vi "GetPanes.vi"(6 "error in":errorcluster, 9 "VI Interpreter in":refnum<class "VI Interpreter.lvclass">) -> (0 "error out":errorcluster, 3 "VI Interpreter out":refnum<class "VI Interpreter.lvclass">, 4 "Panes":refnum<class "Pane.lvclass">[](array[class]))   [LabVIEW 2014, in "VI Interpreter.lvclass"]
uses:
  VI Interpreter.lvclass
  Pane/Pane.lvclass
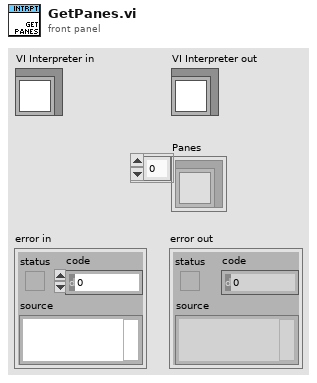
[diagram p1: front panel]
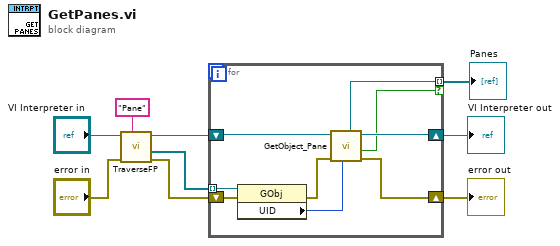
[diagram p0: block diagram]
diagram:
  n1 = call "TraverseFP.vi"("class name"="Pane", "error in"="error in", "VI Interpreter in"="VI Interpreter in") -> ("error out"=w6:errorcluster, "References"=w4:refnum<vi>[], "VI Interpreter out"=w7:refnum<class "VI Interpreter.lvclass">)  [unwired: 4 in]
  n2 = for {
    tunnel: w4 -> [w17] mode=indexing
    shift-right: [w13] -> w9
    shift-left: w7 -> [w18]
    tunnel: [w11] -> w1 mode=indexing if=w10
    shift-right: [w12] -> w2
    shift-left: w6 -> [w16]
    n3 = property class="GObj"(reference=w17, error in=w16) -> (error out=w14:errorcluster, "UID"=w15:i32)  [unwired: 1 out]
    n4 = call "GetObject_Pane.vi"("UID"=w15, "error in"=w14, "VI Interpreter in"=w18) -> ("error out"=w12:errorcluster, "found"=w10:bool, "VI Interpreter out"=w13:refnum<class "VI Interpreter.lvclass">, "pane"=w11:refnum<class "Pane.lvclass">)  [unwired: 3 in]
  }
  "error out" <- w2
  "VI Interpreter out" <- w9
  "Panes" <- w1
